vi "Grid_Main_v11.vi"(10 "Part of multigrid":bool, 11 "Settings":T3={"Drift Correction Settings"={"Drift Correction every"=80, "Drift correction Pixels"=256, "Channel index (0-23)"=0, "MaxImagesBack"=2, "Threshold"=2, "Increment"=8, "max applied Drift Correction"=20, "Correct Drift"=TRUE, "Correlate"=0, "Correct z drift"=FALSE, "zdrift \nDuration (s)"=0.0}, "Spectroscopy Setting"={"Imaging Current"=1e-11, "ref Current"=7e-11, "tip Speed (m/s)"=2e-09, "Imaging Bias"=0.02, "ref Bias"=-0.1, "preSTS delay [ms]"=500, "STS z offset"=2e-10, "during Spec Bias (V)"=-0.1, "trigger1 < Hz"=0.0, "trigger 2 >Hz"=0.0, "autoStop"=FALSE, "Spectroscopy"=0, "PLL ON/OFF"=TRUE, "readjust setpoint every "=1, "z Reference (constHeight)"=FALSE, "Lock In"=TRUE}, "Misc"={"File name"="symmetric_node_zOff=200p", "Email when finished"="cornelius.krull@monash.edu,Dhaneesh.Gopalakrishnan@monash.edu,marina.castelli@monash.edu"}, "Grid Settings"={"type"=1, "type order"=1, "X pixel"=0, "Y pixel"=0, "Grid_Parms"={"center X (m)"=0.0, "center Y (m)"=0.0, "width (m)"=0.0, "height (m)"=0.0, "angle (deg)"=0.0}}} {"Grid Settings"."type order" items=["Grid", "Random", "Adam7"]; "Grid Settings"."type" items=["Line", "Grid", "Cloud"]; "Spectroscopy Setting"."Spectroscopy" items=["Bias", "zSpec"]; "Spectroscopy Setting"."trigger 2 >Hz" format="%#_6p"; "Spectroscopy Setting"."trigger1 < Hz" format="%#_6p"; "Spectroscopy Setting"."during Spec Bias (V)" format="%#_5p"; "Spectroscopy Setting"."STS z offset" format="%#_6p"; "Spectroscopy Setting"."ref Bias" format="%#_6p"; "Spectroscopy Setting"."Imaging Bias" format="%#_6p"; "Spectroscopy Setting"."tip Speed (m/s)" format="%.2p"; "Spectroscopy Setting"."ref Current" format="%#_6p"; "Spectroscopy Setting"."Imaging Current" format="%#_6p"; "Drift Correction Settings"."Correlate" items=["first Frame", "successive Frames"]; "Drift Correction Settings"."max applied Drift Correction" min=1 max=100 step=1 format="%.0p"; "Drift Correction Settings"."Threshold" min=1 step=1; "Drift Correction Settings"."Channel index (0-23)" items=["Current"=0, "Z (m)"=14]}) -> (3 "Settings out":T2)   [LabVIEW 2014]
uses:
  <userlib>/Nanonis Prog Interface V5/Nanonis Prog Interface.lvlib
panel:
  in  "resume":T1
  in  "stop":bool
  out "total points":i32
  out "Points taken":i32
  out "ETA":timestamp=timestamp(3575267058.899443 s since 1904-01-01)
  out "remaining time":dbl format="%<%H:%M:%S>t"
  out "Progress":u8(slide)=100 scale=0.0..100.0 scale format="%#.1g"
  out "Last z adjustment":dbl
  out "Last Drift detected (images back)":i32
  out "Y Offset out":sgl format="%#_6p"
  out "X Offset out":sgl format="%#_6p"
  out "Drift Correction Image":picture
  # "RUN smart tilt before starting the GRID\nCHECK CUTOFF\nmove tip to reference point for tip height"
  # "%"
  # "finish the last action and then"
  # "GRID points"
  # "Increase this if no Drift was detected for \na certain number of images"
  # "% of image size"
  # "Only first frame works"
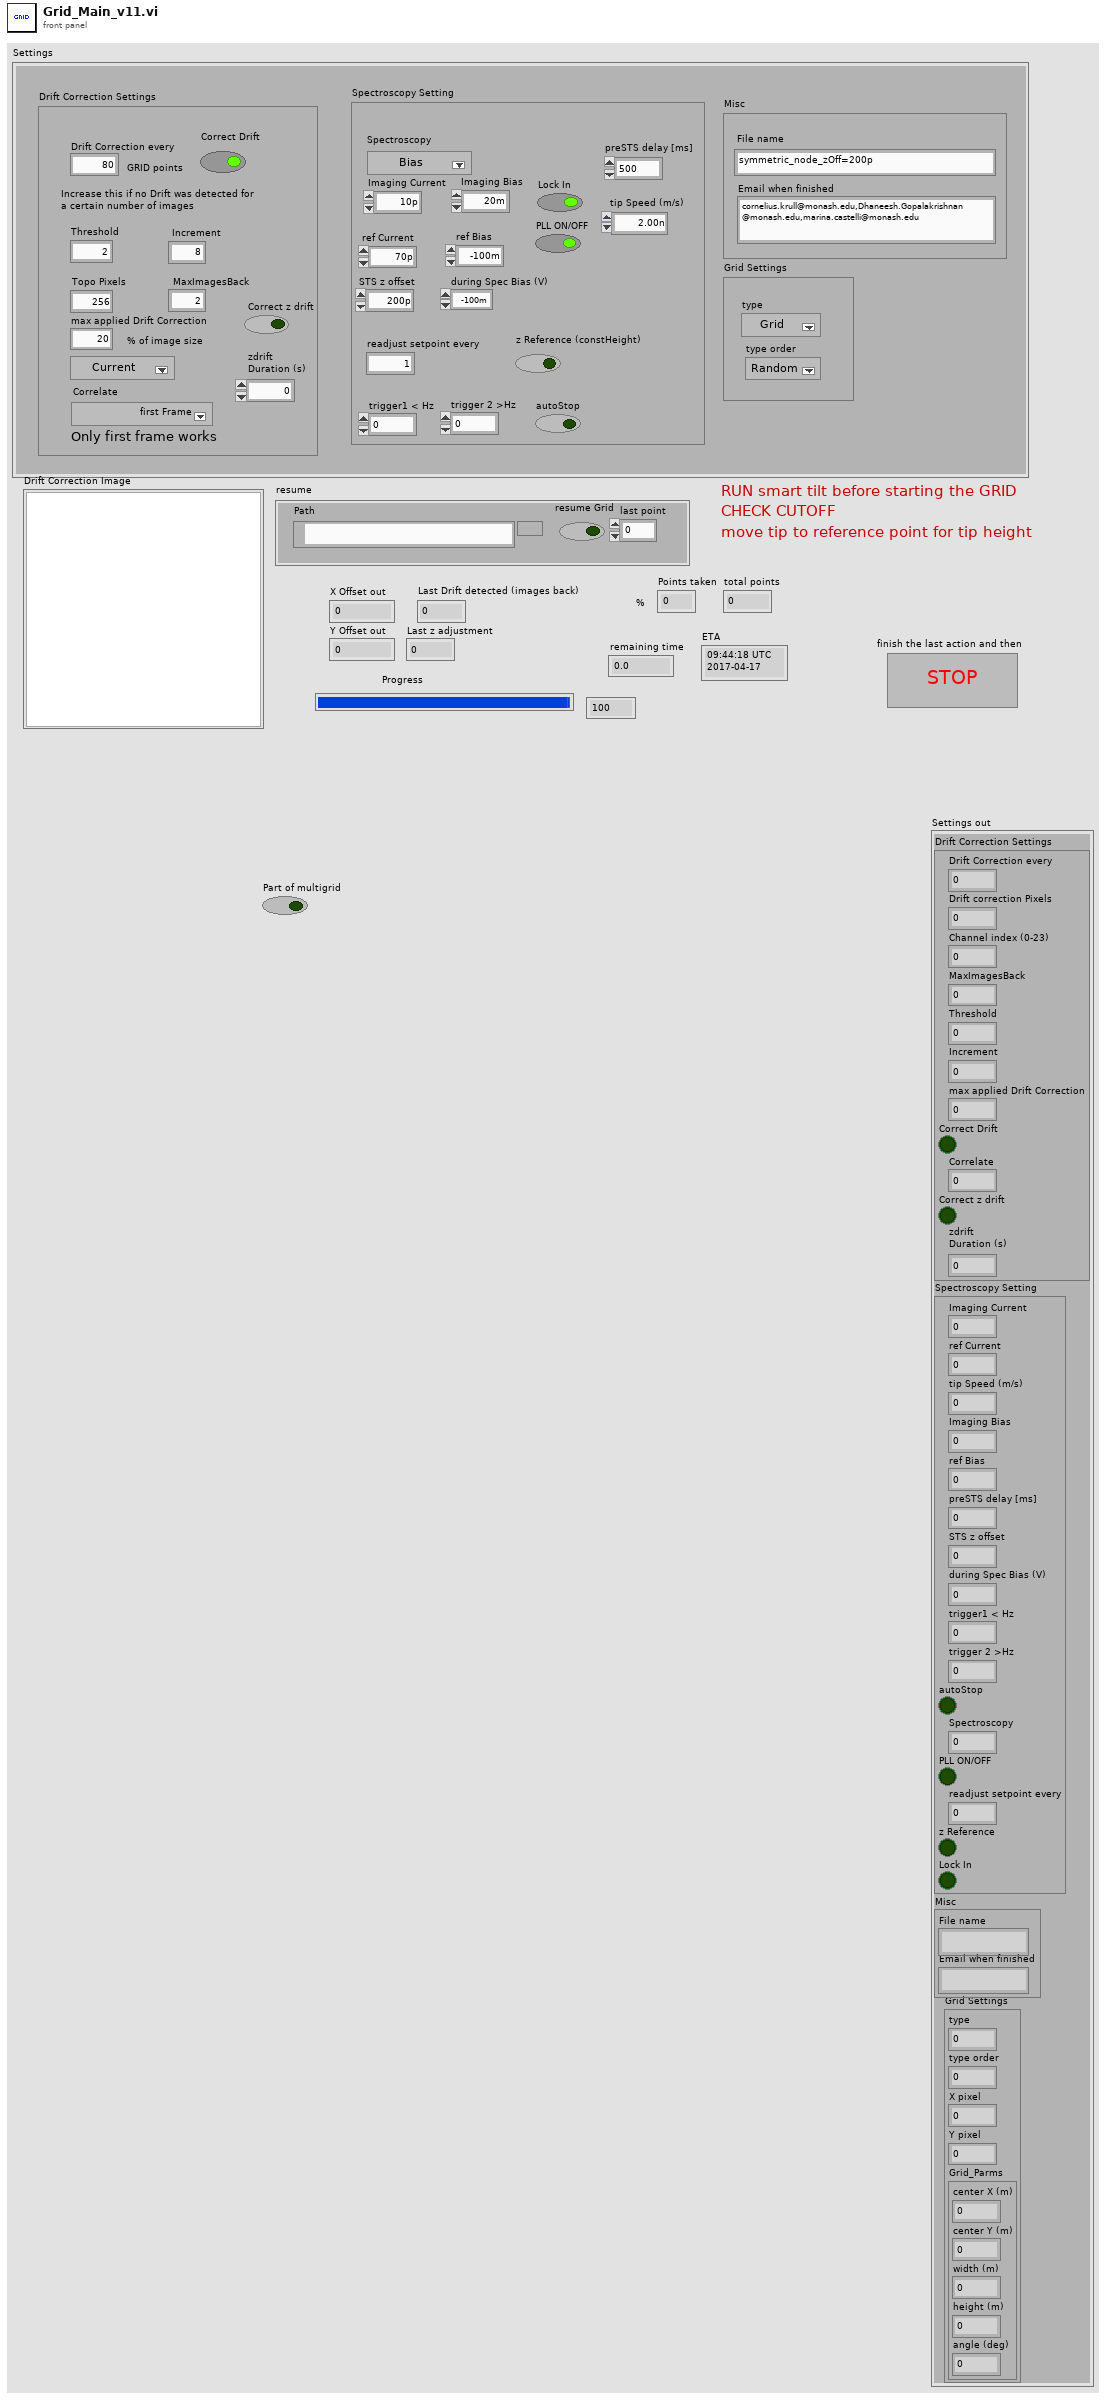
[diagram p1: front panel]
types:
  T1 = cluster{"resume Grid":bool, "Path":path, "last point":i32}
  T2 = cluster{"Drift Correction Settings":cluster{"Drift Correction every":i32, "Drift correction Pixels":i32, "Channel index (0-23)":u8, "MaxImagesBack":i32, "Threshold":i32, "Increment":i32, "max applied Drift Correction":i32, "Correct Drift":bool, "Correlate":u16, "Correct z drift":bool, "zdrift \nDuration (s)":dbl}, "Spectroscopy Setting":cluster{"Imaging Current":dbl, "ref Current":dbl, "tip Speed (m/s)":sgl, "Imaging Bias":dbl, "ref Bias":dbl, "preSTS delay [ms]":u32, "STS z offset":dbl, "during Spec Bias (V)":sgl, "trigger1 < Hz":sgl, "trigger 2 >Hz":sgl, "autoStop":bool, "Spectroscopy":u16, "PLL ON/OFF":bool, "readjust setpoint every ":i32, "z Reference":bool, "Lock In":bool}, "Misc":cluster{"File name":string, "Email when finished":string}, "Grid Settings":cluster{"type":u16, "type order":u16, "X pixel":i32, "Y pixel":i32, "Grid_Parms":cluster{"center X (m)":sgl, "center Y (m)":sgl, "width (m)":sgl, "height (m)":sgl, "angle (deg)":sgl}}}
  T3 = cluster{"Drift Correction Settings":cluster{"Drift Correction every":i32, "Drift correction Pixels":i32, "Channel index (0-23)":u8, "MaxImagesBack":i32, "Threshold":i32, "Increment":i32, "max applied Drift Correction":i32, "Correct Drift":bool, "Correlate":u16, "Correct z drift":bool, "zdrift \nDuration (s)":dbl}, "Spectroscopy Setting":cluster{"Imaging Current":dbl, "ref Current":dbl, "tip Speed (m/s)":sgl, "Imaging Bias":dbl, "ref Bias":dbl, "preSTS delay [ms]":u32, "STS z offset":dbl, "during Spec Bias (V)":sgl, "trigger1 < Hz":sgl, "trigger 2 >Hz":sgl, "autoStop":bool, "Spectroscopy":u16, "PLL ON/OFF":bool, "readjust setpoint every ":i32, "z Reference (constHeight)":bool, "Lock In":bool}, "Misc":cluster{"File name":string, "Email when finished":string}, "Grid Settings":cluster{"type":u16, "type order":u16, "X pixel":i32, "Y pixel":i32, "Grid_Parms":cluster{"center X (m)":sgl, "center Y (m)":sgl, "width (m)":sgl, "height (m)":sgl, "angle (deg)":sgl}}}
  T4 = cluster{"Drift File out":refnum<file>, "zFile":refnum<file>, "BinFile ref":refnum<file>, "xyFile":refnum<file>}
  T5 = cluster{"Drift Correction every":i32, "Drift correction Pixels":i32, "Channel index (0-23)":u8, "MaxImagesBack":i32, "Threshold":i32, "Increment":i32, "max applied Drift Correction":i32, "Correct Drift":bool, "Correlate":u16, "Correct z drift":bool, "zdrift \nDuration (s)":dbl}
  T6 = cluster{"Imaging Current":dbl, "ref Current":dbl, "tip Speed (m/s)":sgl, "Imaging Bias":dbl, "ref Bias":dbl, "preSTS delay [ms]":u32, "STS z offset":dbl, "during Spec Bias (V)":sgl, "trigger1 < Hz":sgl, "trigger 2 >Hz":sgl, "autoStop":bool, "Spectroscopy":u16, "PLL ON/OFF":bool, "readjust setpoint every ":i32, "z Reference":bool, "Lock In":bool}
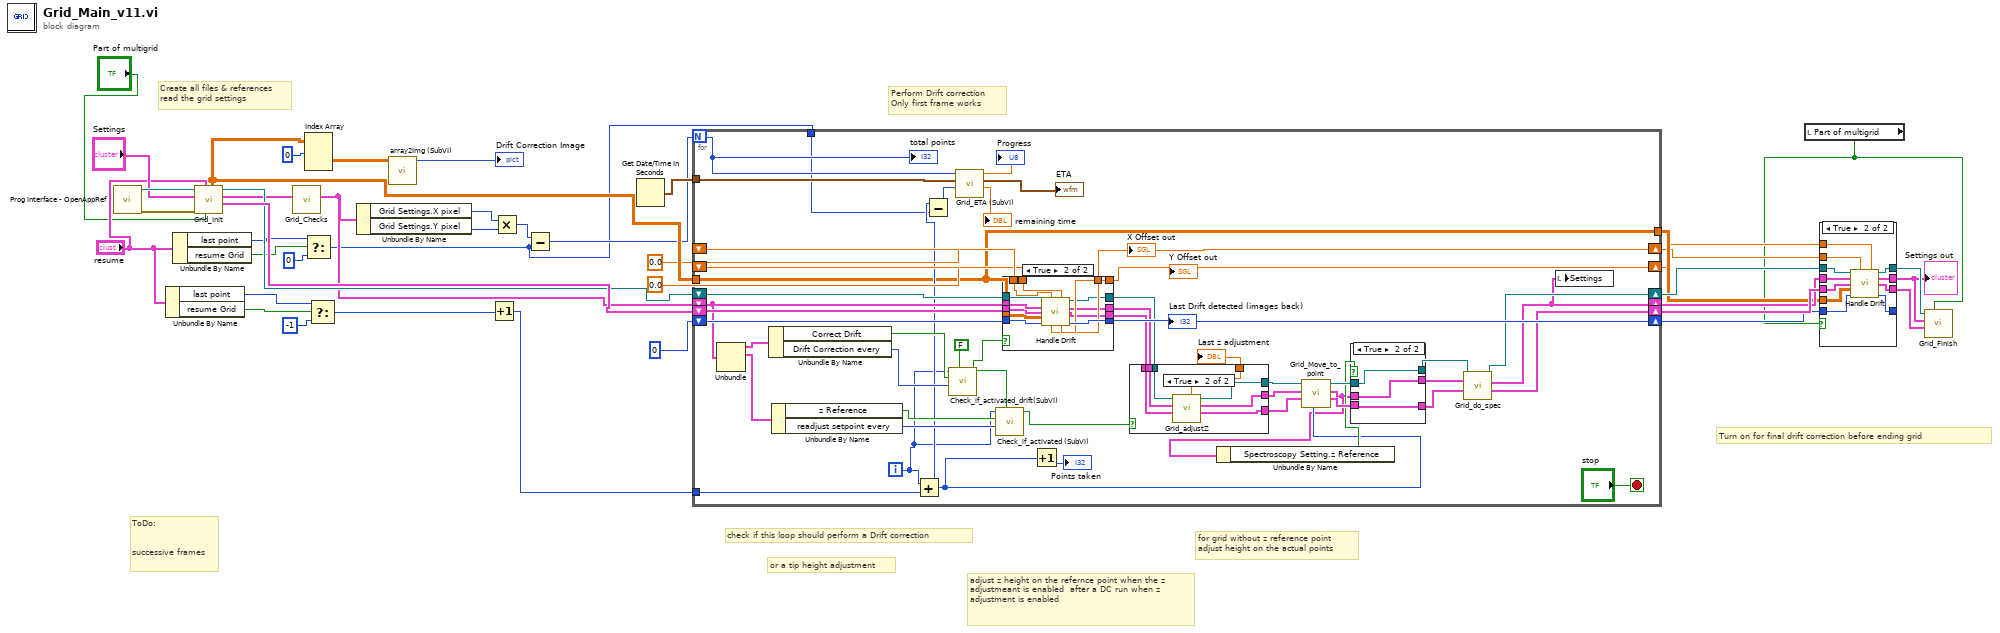
[diagram p0: block diagram]
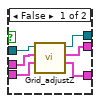
[diagram p3: hidden frame]
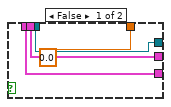
[diagram p4: hidden frame]
diagram:
  # "Turn on for final drift correction before ending grid"
  # "ToDo:\n\n\nsuccessive frames"
  # "Perform Drift correction\nOnly first frame works"
  # "check if this loop should perform a Drift correction"
  # "for grid without z reference point \nadjust height on the actual points"
  # "or a tip height adjustment"
  # "Create all files & references\nread the grid settings"
  # "adjust z height on the refernce point when the z adjustmeant is enabled  after a DC run when z adjustment is enabled"
  n1 = call <userlib>:"Prog Interface - OpenAppRef.vi"() -> ("Error out"=w40:errorcluster, "Application reference"=w41:refnum<vi>)  [unwired: 6 in]
  n2 = Unbundle By Name("resume") -> ("last point"=w22:i32, "resume Grid"=w24:bool)
  n3 = Unbundle By Name("resume") -> ("last point"=w16:i32, "resume Grid"=w18:bool)
  n4 = call "Grid_Init.vi"("Part of multigrid"="Part of multigrid", "resume"="resume", "Error in"=w40, "Settings"="Settings", "Application reference"=w41) -> ("FileRefs"=w38:T4, "Settings out"=w27:T2, "Application ref out"=w37:refnum<vi>, "DC images"=w35:dbl[][][])  [unwired: 2 in, 1 out]
  n5 = call "Grid_Checks.vi"("Settings"=w27) -> ("Settings out"=w26:T2)  [unwired: 10 in]
  n6 = Index Array(array=w35, index (dim 0)=0 ("index (page)")) -> (element=w36:dbl[][])  [unwired: 2 in]
  n7 = Select(t=w16, s=w18, f=0) -> (s? t:f=w13:i32)
  n8 = Select(t=w22, s=w24, f=-1) -> (s? t:f=w21:i32)
  n9 = Unbundle By Name(w26) -> ("Grid Settings.X pixel"=w30:i32, "Grid Settings.Y pixel"=w29:i32)
  n10 = call "array2Img (SubVI).vi"("Rxy"=w36) -> ("new picture"=→"Drift Correction Image":picture)  [unwired: 10 in]
  n11 = Increment(x=w21) -> (x+1=w19:i32)
  n12 = Multiply(x=w30, y=w29) -> (x*y=w14:i32)
  n13 = Subtract(x=w14, y=w13) -> (x-y=w20:i32)
  n14 = Get Date/Time In Seconds() -> (seconds since 1Jan1904=w28:timestamp)
  n15 = for {
    N: w20 -> [w49]
    tunnel: w35 -> [w43]
    shift-right: [w87] -> w8
    shift-left: 0 ("Last Drift out") -> [w86]
    shift-right: [w82] -> w6
    shift-left: sgl 0.0 ("X Offset out") -> [w85]
    shift-right: [w83] -> w5
    shift-left: sgl 0.0 ("Y Offset out") -> [w84]
    tunnel: w28 -> [w73]
    shift-right: [w70] -> w10
    shift-left: w37 -> [w88]
    shift-right: [w45] -> w11
    shift-left: w26 -> [w56]
    shift-right: [w69] -> w12
    shift-left: w38 -> [w89]
    tunnel: w19 -> [w57]
    tunnel: w13 -> [w46]
    tunnel: [w43] -> w7
    i -> [w42]
    stop <- "stop" stop-if-true
    n16 = Unbundle(w56) -> ("Drift Correction Settings"=w55:T5, "Spectroscopy Setting"=w53:T6)  [unwired: 2 out]
    n17 = Unbundle By Name(w55) -> ("Correct Drift"=w54:bool, "Drift Correction every"=w50:i32)
    n18 = Unbundle By Name(w53) -> ("z Reference"=w52:bool, "readjust setpoint every"=w51:i32)
    n19 = Add(x=w42, y=w57) -> (x+y=w47:i32)
    n20 = Subtract(x=w47, y=w46) -> (x-y=w48:i32)
    n21 = call "Check_if_activated_drift(SubVI).vi"("Override"=FALSE, "activate  every  iterations"=w50, "activated?"=w54, "Iteration"=w42) -> ("perform action"=w78:bool)  [unwired: 7 in]
    n22 = call "Grid_ETA (SubVI).vi"("points taken"=w48, "seconds since 1Jan1904"=w73, "points todo"=w49) -> ("Numeric 4"=→"remaining time":dbl, "Time Stamp"=→"ETA":timestamp, "Numeric 3"=→"Progress":dbl)  [unwired: 6 in]
    n23 = call "Check_if_activated (SubVI).vi"("Override"=w78, "activate  every  iterations"=w51, "activated?"=w52, "Iteration"=w42) -> ("perform action"=w79:bool)  [unwired: 7 in]
    n24 = case shown="True" w78 {
      tunnel: w56 -> [w112 w128]
      tunnel: w89 -> [w111 w127]
      tunnel: w88 -> [w110 w126]
      tunnel: w43 -> [_ w125]
      tunnel: [w113 w124] -> w87
      tunnel: w86 -> [w113 w123]
      tunnel: w85 -> [w115 w122]
      tunnel: w84 -> [w114 w121]
      tunnel: [w114 w120] -> w83
      tunnel: [w115 w119] -> w82
      tunnel: [w110 w118] -> w81
      tunnel: [w112 w117] -> w59
      tunnel: [w111 w116] -> w80
      frame False {
      }
      frame True {
        n25 = call "Handle Drift.vi"("Application ref in"=w126, "X Offset in"=w122, "Y Offset In"=w121, "Settings"=w128, "FileRefs"=w127, "Drift Correction image"=w125, "Last Drift"=w123) -> ("Application out"=w118:refnum<vi>, "Settings out"=w117:T2, "FileRefs out File Refs  Out"=w116:T4, "X Offset out"=w119:sgl, "Y Offset out"=w120:sgl, "Last Drift out"=w124:i32)  [unwired: 3 in]
      }
    }
    "X Offset out" <- w82
    "Y Offset out" <- w83
    "Last Drift detected (images back)" <- w87
    n26 = Increment(x=w47) -> (x+1=→"Points taken":i32)
    n27 = case shown="True" w79 {
      tunnel: w81 -> [w101 w109]
      tunnel: w80 -> [w100 w108]
      tunnel: w59 -> [w99 w107]
      tunnel: [w100 w106] -> w72
      tunnel: [w99 w105] -> w61
      tunnel: [w101 w104] -> w71
      tunnel: [0.0 ("Last z adjustment") w103] -> w68
      frame False {
      }
      frame True {
        n28 = call "Grid_adjustZ.vi"("FileRefs"=w108, "Settings"=w107, "Application in"=w109) -> ("FileRefs out"=w106:T4, "Settings out"=w105:T2, "Application ref out"=w104:refnum<vi>, "Last z adjustment"=w103:dbl)  [unwired: 4 in, 1 out]
      }
    }
    "Last z adjustment" <- w68
    n29 = call "Grid_Move_to_point.vi"("point"=w47, "FileRefs in"=w72, "Settings"=w61, "Application ref in"=w71) -> ("FileRefs out"=w63:T4, "Settings out"=w44:T2, "Application ref out"=w64:refnum<vi>)  [unwired: 5 in]
    n30 = Unbundle By Name(w44) -> ("Spectroscopy Setting.z Reference"=w62:bool)
    n31 = case shown="True" w62 {
      tunnel: [w95 w98] -> w67
      tunnel: [w94 w96] -> w65
      tunnel: [w93 w97] -> w66
      tunnel: w64 -> [w92 w98]
      tunnel: w44 -> [w91 w97]
      tunnel: w63 -> [w90 w96]
      frame False {
        n32 = call "Grid_adjustZ.vi"("FileRefs"=w90, "Settings"=w91, "Application in"=w92) -> ("FileRefs out"=w94:T4, "Settings out"=w93:T2, "Application ref out"=w95:refnum<vi>)  [unwired: 4 in, 2 out]
      }
      frame True {
      }
    }
    n33 = call "Grid_do_spec.vi"("FileRefs in"=w65, "Settings in"=w66, "Application ref in"=w67) -> ("FileRefs out"=w69:T4, "Settings out"=w45:T2, "Application ref out"=w70:refnum<vi>)  [unwired: 5 in, 1 out]
    n34 = local write "Settings"(w45) -> ()
    "total points" <- w49
  }
  n35 = local read "Part of multigrid"() -> (w2:bool)
  n36 = case shown="True" w2 {
    tunnel: w11 -> [w131 w143]
    tunnel: w12 -> [w130 w142]
    tunnel: w10 -> [w129 w141]
    tunnel: [w132 w140] -> _
    tunnel: w8 -> [w132 w136]
    tunnel: [w129 w139] -> w9
    tunnel: [w131 w138] -> w3
    tunnel: [w130 w137] -> w4
    tunnel: w7 -> [_ w135]
    tunnel: w6 -> [_ w134]
    tunnel: w5 -> [_ w133]
    frame False {
    }
    frame True {
      n37 = call "Handle Drift.vi"("Application ref in"=w141, "X Offset in"=w134, "Y Offset In"=w133, "Settings"=w143, "FileRefs"=w142, "Drift Correction image"=w135, "Last Drift"=w136) -> ("Application out"=w139:refnum<vi>, "Settings out"=w138:T2, "FileRefs out File Refs  Out"=w137:T4, "Last Drift out"=w140:i32)  [unwired: 3 in, 2 out]
    }
  }
  "Settings out" <- w3
  n38 = call "Grid_Finish.vi"("Part of multigrid"=w2, "FileRefs"=w4, "Settings"=w3, "Application reference"=w9) -> ()  [unwired: 8 in]
